vi "注册账号.vi"() -> ()   [LabVIEW 2018]
panel:
  in  "确定按钮":bool
  out "当前时间":timestamp
  out "显示验证码":string
  in  "验证码":string
  out "布尔":bool
  in  "文件路径（使用对话框） 2":path=path "D:/Labviewprogram/登录界面/密码.txt"
  in  "文件路径（使用对话框）":path=path "D:/Labviewprogram/登录界面/账户.txt"
  in  "确认密码":string
  in  "密码":string
  in  "账户":string
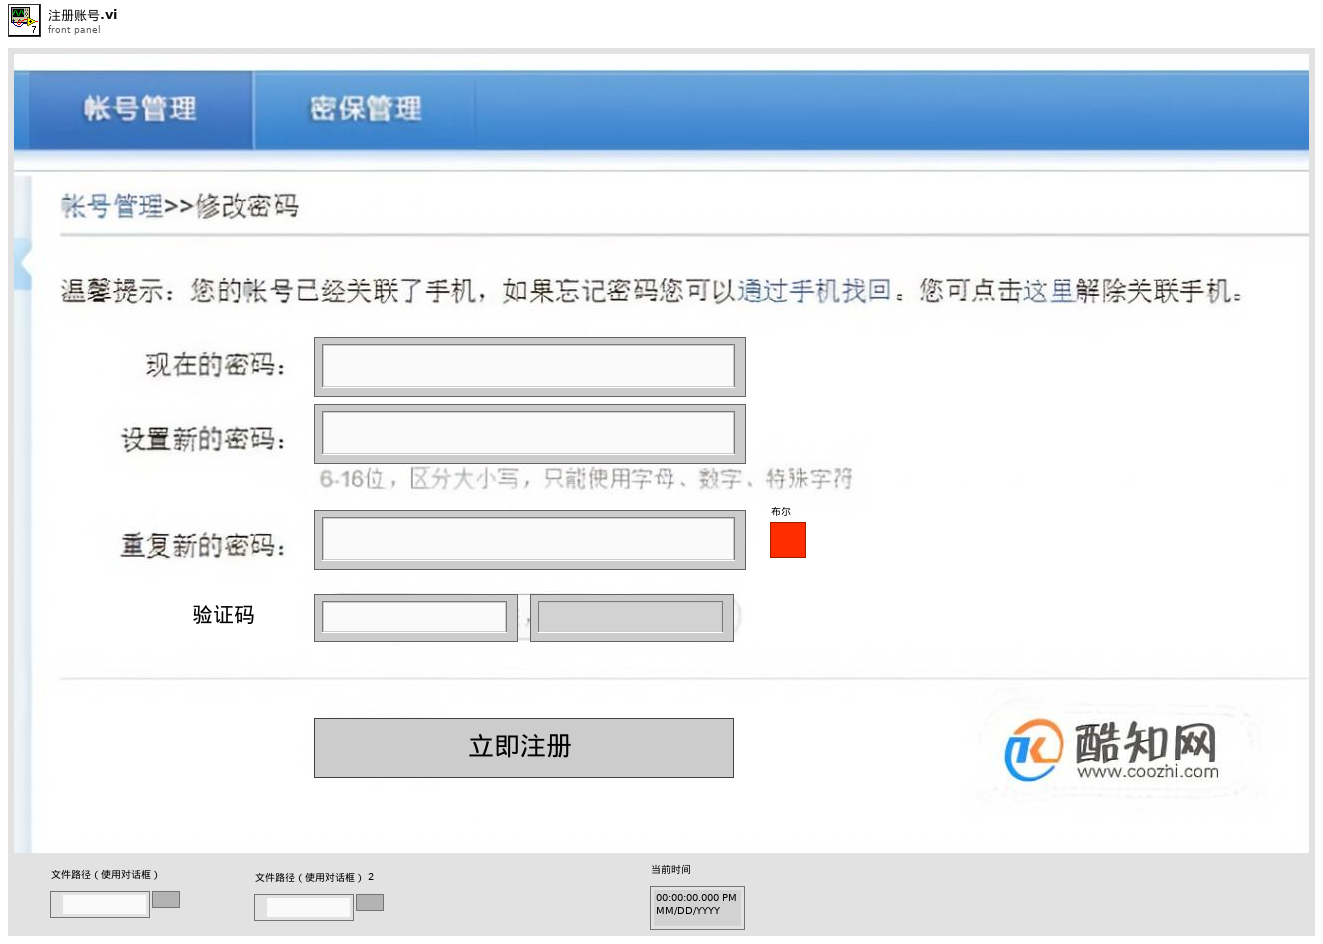
[diagram p1: front panel]
types:
  T1 = enum16{"open", "replace", "create", "open or create", "replace or create", "replace or create with confirmation"}
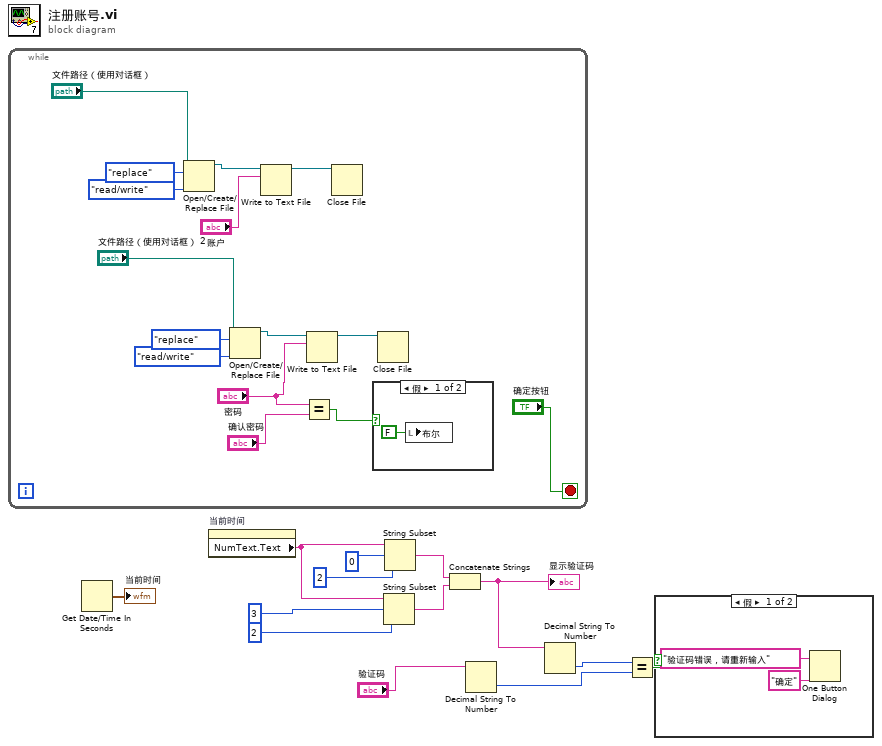
[diagram p0: block diagram]
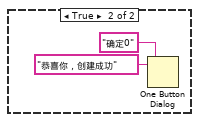
[diagram p2: hidden frame]
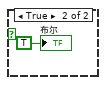
[diagram p3: hidden frame]
diagram:
  n1 = while {
    stop <- "确定按钮" stop-if-true
    n2 = Open/Create/Replace File(file path (use dialog)="文件路径（使用对话框）", operation (0:open)=T1."replace" ("操作(0:open)"), access (0:read/write)=enum16{"read/write", "read-only", "write-only"}."read/write" ("权限(0:read/write)")) -> (refnum out=w28:refnum<file>)  [unwired: 3 in, 2 out]
    n3 = Open/Create/Replace File(file path (use dialog)="文件路径（使用对话框） 2", operation (0:open)=T1."replace" ("操作(0:open)"), access (0:read/write)=enum16{"read/write", "read-only", "write-only"}."read/write" ("权限(0:read/write)")) -> (refnum out=w18:refnum<file>)  [unwired: 3 in, 2 out]
    n4 = Write to Text File(file (use dialog)=w28, text="账户") -> (refnum out=w27:refnum<file>)  [unwired: 2 in, 2 out]
    n5 = Equal?(x="密码", y="确认密码") -> (x = y?=w15:bool)
    n6 = Write to Text File(file (use dialog)=w18, text="密码") -> (refnum out=w19:refnum<file>)  [unwired: 2 in, 2 out]
    n7 = Close File(refnum=w27) -> ()  [unwired: 1 in, 2 out]
    n8 = case shown="假" w15 {
      frame False {
        n9 = local write "布尔"(FALSE ("布尔")) -> ()
      }
      frame True {
        "布尔" <- TRUE ("布尔")
      }
    }
    n10 = Close File(refnum=w19) -> ()  [unwired: 1 in, 2 out]
  }
  n11 = Get Date/Time In Seconds() -> (seconds since 1Jan1904=→"当前时间":timestamp)
  n12 = property on="当前时间" class="AbsTime (严格)"() -> ("NumText.Text"=w10:string)  [unwired: 2 in, 2 out]
  n13 = String Subset(string=w10, offset (0)=3 ("偏移量(0)"), length (rest)=2 ("长度（剩余）")) -> (substring=w6:string)
  n14 = String Subset(string=w10, offset (0)=0 ("偏移量(0)"), length (rest)=2 ("长度（剩余）")) -> (substring=w7:string)
  n15 = Concatenate Strings(w7, w6) -> (w5:string)
  "显示验证码" <- w5
  n16 = Decimal String To Number(string="验证码") -> (number=w2:i32)  [unwired: 2 in, 1 out]
  n17 = Decimal String To Number(string=w5) -> (number=w3:i32)  [unwired: 2 in, 1 out]
  n18 = Equal?(x=w3, y=w2) -> (x = y?=w1:bool)
  n19 = case shown="假" w1 {
    frame False {
      n20 = One Button Dialog(message="验证码错误，请重新输入" ("消息"), button name ("OK")="确定" ("按钮名称（“确定”）")) -> ()  [unwired: 1 out]
    }
    frame True {
      n21 = One Button Dialog(message="恭喜你，创建成功" ("消息"), button name ("OK")="确定0" ("按钮名称（“确定”）")) -> ()  [unwired: 1 out]
    }
  }
